vi "day 1 task 1.vi"() -> ()   [LabVIEW 2019]
panel:
  out "no. calories carried by elf with most":i32
  out "sorted array (large to small)":i32[](array[numeric])
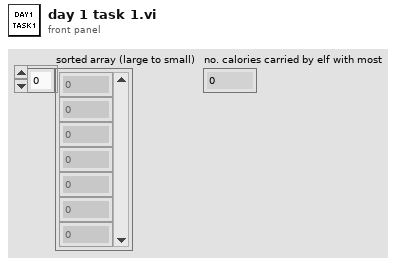
[diagram p1: front panel]
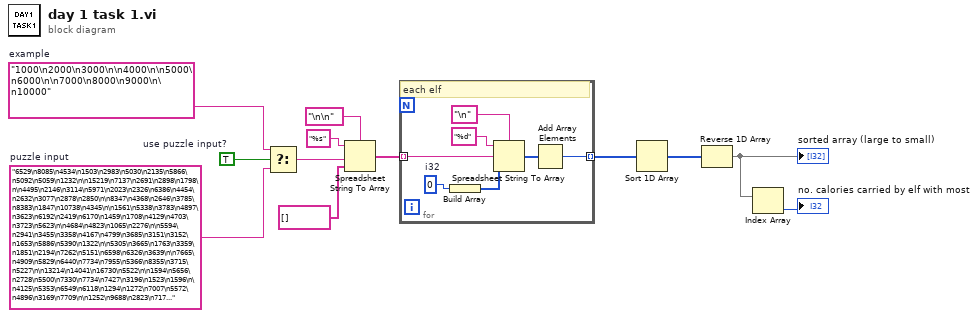
[diagram p0: block diagram]
diagram:
  w2 = TRUE  # use puzzle input?
  w3 = "6529\n8085\n4534\n1503\n2983\n5030\n2135\n5866\n5092\n5059\n1232\n\n15219\n7137\n2691\n2898\n1798\n\n4495\n2146\n3114\n5971\n2023\n2326\n6386\n4454\n2632\n3077\n2878\n2850\n\n8347\n4368\n2646\n3785\n8383\n1847\n10738\n4345\n\n1561\n5338\n3783\n4897\n3623\n6192\n2419\n6170\n1459\n1708\n4129\n4703\n3723\n5623\n\n4684\n4823\n1065\n2276\n\n5594\n2941\n3455\n3358\n4167\n4799\n3685\n3151\n3152\n1653\n5886\n5390\n1322\n\n5305\n3665\n1763\n3359\n1851\n2194\n7262\n5151\n6598\n6326\n3639\n\n7665\n4909\n5829\n6440\n7734\n7955\n5366\n8355\n3715\n5227\n\n13214\n14041\n16730\n5522\n\n1594\n5656\n2728\n5500\n7330\n7734\n7427\n3196\n1523\n1596\n\n4125\n5353\n6549\n6118\n1294\n1272\n7007\n5572\n4896\n3169\n7709\n\n1252\n9688\n2823\n717..."  # puzzle input
  w4 = "1000\n2000\n3000\n\n4000\n\n5000\n6000\n\n7000\n8000\n9000\n\n10000"  # example
  n1 = Select(t=w4, s=w2, f=w3) -> (s? t:f=w1:string)
  n2 = Spreadsheet String To Array(delimiter (Tab)="\n\n", format string="%s", spreadsheet string=w1, array type (2D Dbl)=string[] []) -> (array=w9:string[])
  n3 = for {
    tunnel: w9 -> [w15] mode=indexing
    tunnel: [w13] -> w8 mode=indexing
    w16 = 0  # i32
    # "each elf"
    n4 = Build Array(w16) -> (w17:i32[])
    n5 = Spreadsheet String To Array(delimiter (Tab)="\n", format string="%d", spreadsheet string=w15, array type (2D Dbl)=w17) -> (array=w14:i32[])
    n6 = Add Array Elements(numeric array=w14) -> (sum=w13:i32)
  }
  n7 = Sort 1D Array(array=w8) -> (sorted array=w7:i32[])
  n8 = Reverse 1D Array(array=w7) -> (reversed array=w6:i32[])
  "sorted array (large to small)" <- w6
  n9 = Index Array(array=w6) -> (element=→"no. calories carried by elf with most":i32)  [unwired: 1 in]
